vi "Change Extension - Copy.vi"() -> ()   [LabVIEW 2011]
panel:
  out "concatenated string":string
  in  "Name of File":string
  in  "path":path
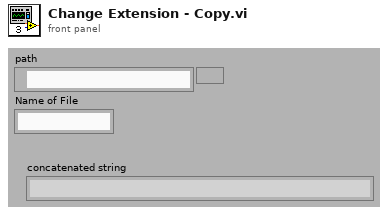
[diagram p1: front panel]
types:
  T1 = enum16{"open", "replace", "create", "open or create", "replace or create", "replace or create with confirmation"}
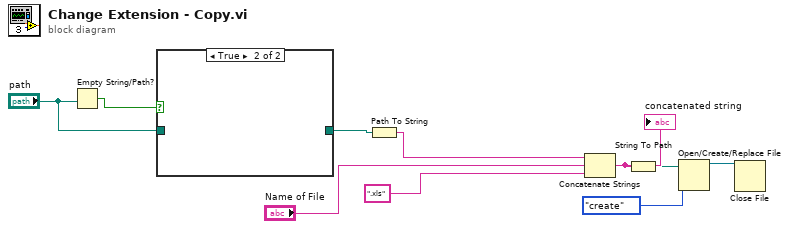
[diagram p0: block diagram]
diagram:
  n1 = Empty String/Path?(string/path="path") -> (empty?=w10:bool)
  n2 = case shown="True" w10 {
    tunnel: [w11 _] -> w9
    tunnel: "path" -> [w11 _]
    frame False {
    }
    frame True {
    }
  }
  n3 = Path To String(path=w9) -> (string=w7:string)
  n4 = Concatenate Strings(w7, "Name of File", ".xls" ("string")) -> (w4:string)
  "concatenated string" <- w4
  n5 = String To Path(string=w4) -> (path=w3:path)
  n6 = Open/Create/Replace File(file path (use dialog)=w3, operation (0:open)=T1."create") -> (refnum out=w1:refnum<file>)  [unwired: 4 in, 2 out]
  n7 = Close File(refnum=w1) -> ()  [unwired: 1 in, 2 out]
